vi "testIsTelQueueToDdsFull.vi"(8 "error in (no error)":errorcluster) -> (0 "error out":errorcluster)   [LabVIEW 2018]
doc: "Test the IsTcpClientQueueFull.vi with queueToDds option."
uses:
  src/TcpServer/TcpServer.lvclass
  src/TcpServerTel/typedef/telTypeDef.ctl
  src/TcpServerTel/typedef/queueOptionsTypeDef.ctl
  src/TcpServerTel/typedef/enqueueOptionsTypeDef.ctl
  src/TcpServer/configServerTypeDef.ctl
  src/TcpServer/TcpServer.lvclass/TcpServer.ctl
  src/TcpServerBase/TcpServerBase.lvclass/TcpServerBase.ctl
  src/TcpServerTel/TcpServerTel.lvclass
  home/pcortes/github/ts_labview_tcp_json/src/TcpServerBase/TcpServerBase.lvclass
  <vilib>/addons/_JKI Toolkits/Caraya/classes/Assert/Assert False.vi
  <vilib>/addons/_JKI Toolkits/Caraya/classes/Assert/Assert True.vi
  <vilib>/addons/_JKI Toolkits/Caraya/classes/Test/Test.lvclass
  <vilib>/addons/_JKI Toolkits/Caraya/classes/Assert/Assert.lvclass
  src/TcpServerBase/TcpServerBase.lvclass
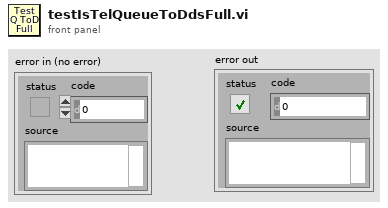
[diagram p1: front panel]
types:
  T1 = enum16{"queueTcpClientFromDds", "queueTcpClient"}
  T2 = typedef "TcpServer.lvclass/configServerTypeDef.ctl" = cluster{"cmdServerPort":u16, "telServerPort":u16, "timeoutServerInMs":i32, "serverBytesToRead":i32, "maxSizeQueueTcpClientFromDds":i32, "EnqueueOptions":T3, "timeoutQueueTcpClientFromDds (ms)":i32, "maxSizeQueueTcpClient":i32, "timeoutInMs":i32}
  T3 = typedef "TcpServerTel.lvclass/enqueueOptionsTypeDef.ctl" = enum16{"lossy enqueue", "normal enqueue"}
  T4 = typedef "TcpServerTel.lvclass/queueOptionsTypeDef.ctl" = cluster{"EnqueueOptions":T3, "Timeout (ms)":i32}
  T5 = typedef "TcpServerTel.lvclass/telTypeDef.ctl" = cluster{"name":string, "telDetails":string}
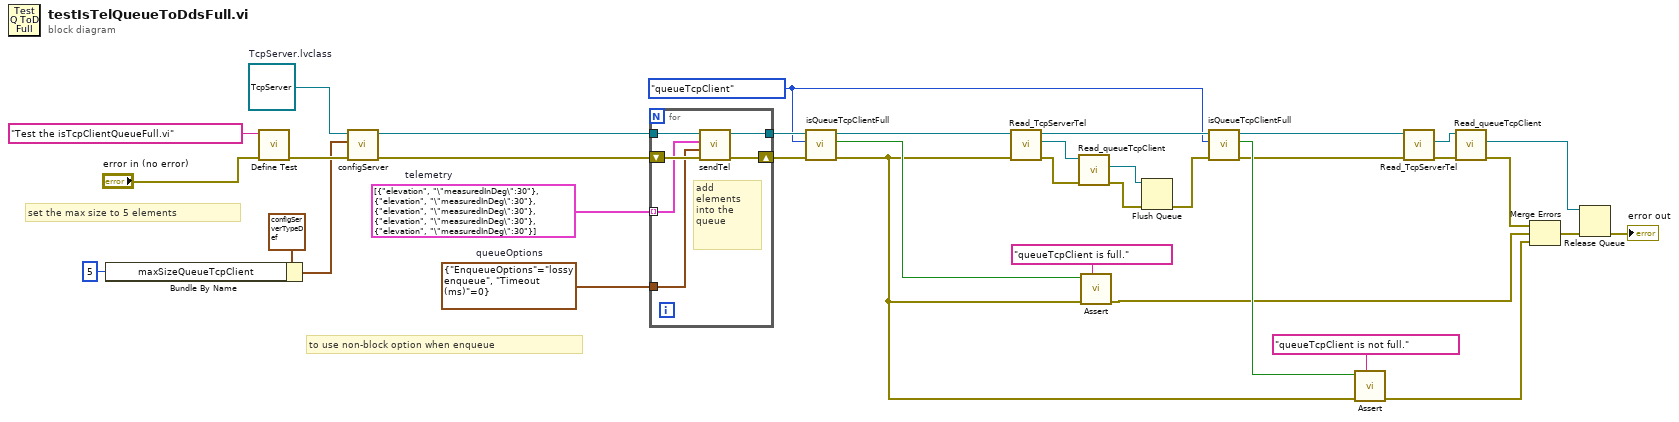
[diagram p0: block diagram]
diagram:
  w1 = T1."queueTcpClient" ("queueName")
  w4 = T4 {"EnqueueOptions"=enum."lossy enqueue", "Timeout (ms)"=0}  # queueOptions
  w5 = T5[] [{"name"="elevation", "telDetails"="\"measuredInDeg\":30"}, {"name"="elevation", "telDetails"="\"measuredInDeg\":30"}, {"name"="elevation", "telDetails"="\"measuredInDeg\":30"}, {"name"="elevation", "telDetails"="\"measuredInDeg\":30"}, {"name"="elevation", "telDetails"="\"measuredInDeg\":30"}]  # telemetry
  w25 = refnum<class "TcpServer.lvclass"> refnum  # TcpServer.lvclass
  # "to use non-block option when enqueue"
  # "set the max size to 5 elements"
  n1 = Bundle By Name(cluster=T2 {"cmdServerPort"=8888, "telServerPort"=8889, "timeoutServerInMs"=100, "serverBytesToRead"=32768, "maxSizeQueueTcpClientFromDds"=1000, "EnqueueOptions"=enum."lossy enqueue", "timeoutQueueTcpClientFromDds (ms)"=50, "maxSizeQueueTcpClient"=1000, "timeoutInMs"=100} ("ServerConfiguration"), "maxSizeQueueTcpClient"=5 ("telQueueServerMaxSize")) -> (w3:T2)
  n2 = call <vilib>:"Define Test.vi"("error in (no error)"="error in (no error)", "Label (VI Title)"="Test the isTcpClientQueueFull.vi") -> ("error out"=w24:errorcluster)  [unwired: 9 in]
  n3 = call "configServer.vi"("error in (no error)"=w24, "ServerConfiguration"=w3, "tcpServer in"=w25) -> ("error out"=w23:errorcluster, "tcpServer out"=w7:refnum<class "TcpServer.lvclass">)  [unwired: 7 in]
  n4 = for {
    shift-right: [w41] -> w22
    shift-left: w23 -> [w42]
    tunnel: w7 -> [w40]
    tunnel: [w39] -> w6
    tunnel: w5 -> [w38] mode=indexing
    tunnel: w4 -> [w37]
    # "add \nelements\ninto the \nqueue"
    n5 = call "sendTel.vi"("error in (no error)"=w42, "queueOptions"=w37, "Telemetry"=w38, "tcpServer in"=w40) -> ("error out"=w41:errorcluster, "tcpServer out"=w39:refnum<class "TcpServer.lvclass">)  [unwired: 6 in]
  }
  n6 = call "isQueueTcpClientFull.vi"("error in (no error)"=w22, "queueName"=w1, "tcpServer in"=w6) -> ("error out"=w13:errorcluster, "queueFull"=w31:bool, "tcpServer out"=w19:refnum<class "TcpServer.lvclass">)  [unwired: 6 in]
  n7 = call "Read_TcpServerTel.vi"("error in (no error)"=w13, "TcpServer in"=w19) -> ("error out"=w20:errorcluster, "TcpServerTel.lvclass"=w21:refnum<class "TcpServerTel.lvclass">, "TcpServer out"=w16:refnum<class "TcpServer.lvclass">)  [unwired: 7 in]
  n8 = call "Read_queueTcpClient.vi"("error in (no error)"=w20, "TcpServerBase in"=w21) -> ("error out"=w17:errorcluster, "queueTcpClient"=w18:refnum<queue>)  [unwired: 7 in, 1 out]
  n9 = call-poly <vilib>:"Assert.vi"("Label"="queueTcpClient is full.", "error in (no error)"=w13, "True?"=w31) -> ("error out"=w9:errorcluster)  [unwired: 8 in]
  n10 = Flush Queue(queue=w18, error in (no error)=w17) -> (error out=w15:errorcluster)  [unwired: 2 out]
  n11 = call "isQueueTcpClientFull.vi"("error in (no error)"=w15, "queueName"=w1, "tcpServer in"=w16) -> ("error out"=w10:errorcluster, "queueFull"=w12:bool, "tcpServer out"=w11:refnum<class "TcpServer.lvclass">)  [unwired: 6 in]
  n12 = call-poly <vilib>:"Assert.vi"("Label"="queueTcpClient is not full.", "error in (no error)"=w13, "False?"=w12) -> ("error out"=w8:errorcluster)  [unwired: 8 in]
  n13 = call "Read_TcpServerTel.vi"("error in (no error)"=w10, "TcpServer in"=w11) -> ("error out"=w30:errorcluster, "TcpServerTel.lvclass"=w29:refnum<class "TcpServerTel.lvclass">)  [unwired: 7 in, 1 out]
  n14 = call "Read_queueTcpClient.vi"("error in (no error)"=w30, "TcpServerBase in"=w29) -> ("error out"=w27:errorcluster, "queueTcpClient"=w28:refnum<queue>)  [unwired: 7 in, 1 out]
  n15 = Merge Errors(w27, w9, w8) -> (w32:errorcluster)
  n16 = Release Queue(queue=w28, error in (no error)=w32) -> (error out=→"error out":errorcluster)  [unwired: 1 in, 2 out]
